vi "MarkBoardPerimeter.vi"(11 "Board In":bool[][](array[boolean])) -> (3 "Board With Perimeter":bool[][](array[boolean]))   [LabVIEW 2015, in "TronVIEWGameUtilities.lvlib"]
uses:
  TronVIEWGameUtilities.lvlib
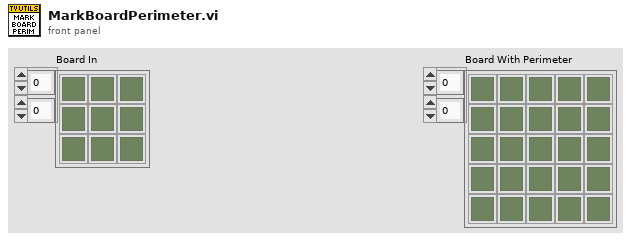
[diagram p1: front panel]
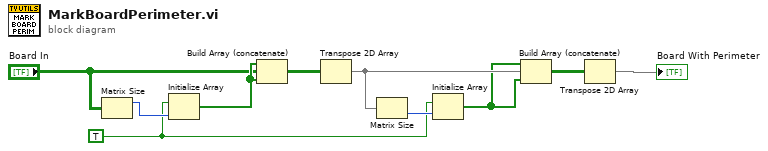
[diagram p0: block diagram]
diagram:
  w1 = TRUE
  n1 = Matrix Size(0:"Board In") -> (1:w10:i32)  [unwired: 1 out]
  n2 = Initialize Array(w1, w10) -> (w8:bool[])
  n3 = Build Array (concatenate)(w8, "Board In", w8) -> (w9:bool[][])
  n4 = Transpose 2D Array(2D array=w9) -> (transposed array=w6:bool[][])
  n5 = Matrix Size(0:w6) -> (2:w4:i32)  [unwired: 1 out]
  n6 = Initialize Array(w1, w4) -> (w5:bool[])
  n7 = Build Array (concatenate)(w5, w6, w5) -> (w7:bool[][])
  n8 = Transpose 2D Array(2D array=w7) -> (transposed array=→"Board With Perimeter":bool[][])
